vi "32_7_matrix_inverse.vi"(2 "n":i32, 3 "A":fxp<+/-,32,7>[](array[numeric])) -> (0 "divide by zero detected":bool, 1 "inv(A)":fxp<+/-,32,7>[](array[numeric]))   [LabVIEW 2020]
panel:
  in  "FXP_3":fxp<+,32,7>
  in  "FXP_2":fxp<+/-,32,7>=1.0 format="%#_32g"
  in  "FXP_1":fxp<+/-,32,7>
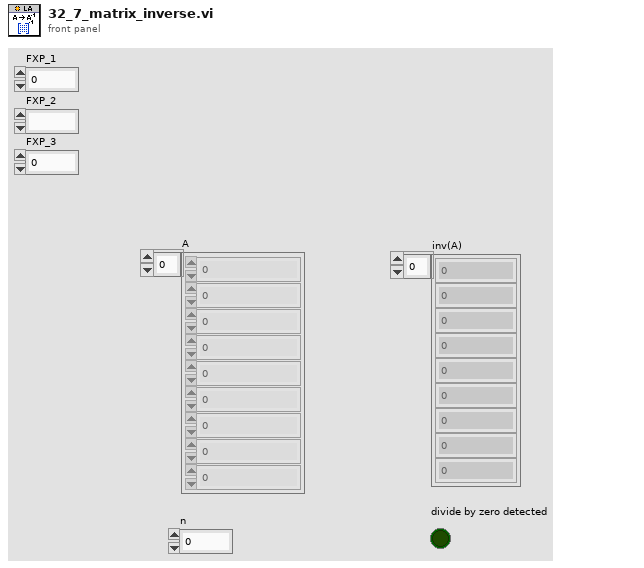
[diagram p1: front panel]
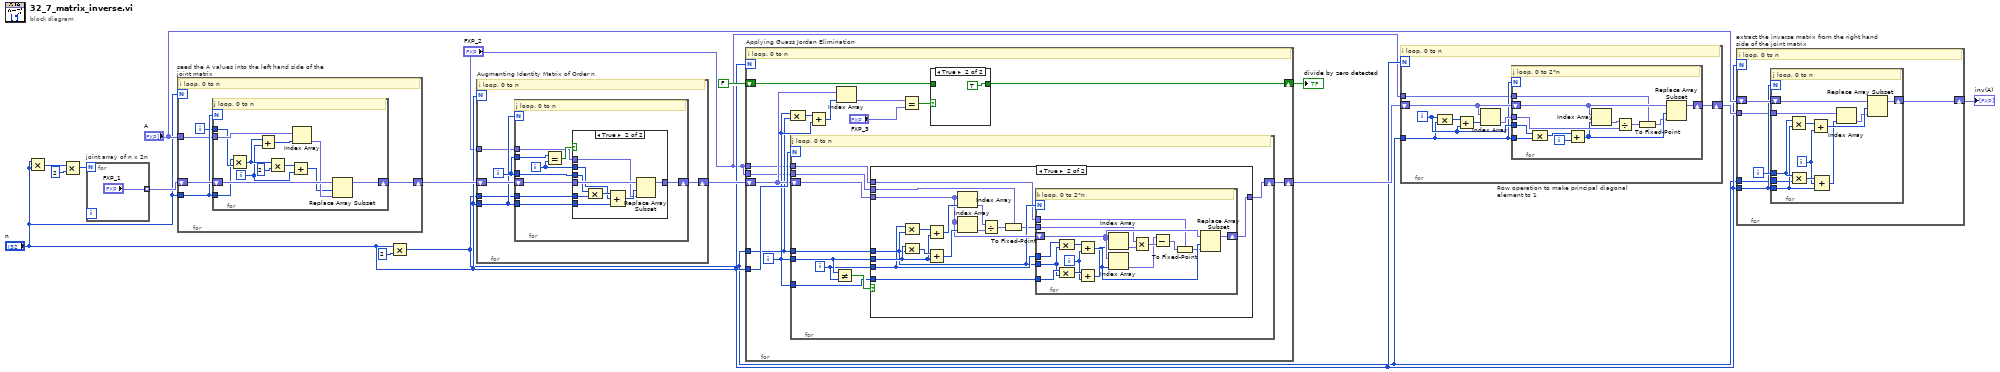
[diagram p0: block diagram]
diagram:
  n1 = Multiply(x="n", y="n") -> (x*y=w3:i32)
  n2 = Multiply(x=w3, y=2) -> (x*y=w6:i32)
  n3 = for "joint array of n x 2n" {
    N: w6 -> [_]
    tunnel: ["FXP_1"] -> w7 mode=indexing
  }
  n4 = for "seed the A values into the left hand side of the joint matrix" {
    N: "n" -> [_]
    shift-right: [w21] -> w8
    shift-left: w7 -> [w22]
    tunnel: "n" -> [w20]
    tunnel: "A" -> [w19]
    i -> [w18]
    # "i loop, 0 to n"
    n5 = for {
      N: w20 -> [_]
      shift-right: [w33] -> w21
      shift-left: w22 -> [w34]
      tunnel: w20 -> [w30]
      tunnel: w19 -> [w32]
      tunnel: w18 -> [w31]
      i -> [w24]
      # "j loop, 0 to n"
      n6 = Multiply(x=w30, y=w31) -> (x*y=w26:i32)
      n7 = Add(x=w26, y=w24) -> (x+y=w29:i32)
      n8 = Multiply(x=w26, y=2) -> (x*y=w25:i32)
      n9 = Add(x=w25, y=w24) -> (x+y=w23:i32)
      n10 = Index Array(array=w32, index=w29) -> (element=w28:fxp<+/-,32,7>)
      n11 = Replace Array Subset(array=w34, new element=w28, index=w23) -> (w33:fxp<+/-,32,7>[])
    }
  }
  n12 = Multiply(x="n", y=2) -> (x*y=w2:i32)
  n13 = for "Augmenting Identity Matrix of Order n" {
    N: "n" -> [_]
    shift-right: [w39] -> w11
    shift-left: w8 -> [w40]
    tunnel: "n" -> [w37]
    tunnel: w2 -> [w36]
    tunnel: "FXP_2" -> [w35]
    i -> [w38]
    # "i loop, 0 to n"
    n14 = for {
      N: w37 -> [_]
      tunnel: w38 -> [w49]
      shift-right: [w46] -> w39
      shift-left: w40 -> [w47]
      tunnel: w38 -> [w45]
      tunnel: w37 -> [w44]
      tunnel: w36 -> [w42]
      tunnel: w35 -> [w41]
      i -> [w43]
      # "j loop, 0 to n"
      n15 = Equal?(x=w49, y=w43) -> (x = y?=w48:bool)
      n16 = case shown="True" w48 {
        tunnel: w47 -> [w50 w59]
        tunnel: [w50 w57] -> w46
        tunnel: w45 -> [_ w58]
        tunnel: w44 -> [_ w54]
        tunnel: w43 -> [_ w55]
        tunnel: w42 -> [_ w52]
        tunnel: w41 -> [_ w51]
        frame False {
        }
        frame True {
          n17 = Compound Arithmetic op=MULTIPLY(w58, w52) -> (w56:i32)
          n18 = Compound Arithmetic op=ADD(w56, w55, w54) -> (w53:i32)
          n19 = Replace Array Subset(array=w59, new element=w51, index=w53) -> (w57:fxp<+/-,32,7>[])
        }
      }
    }
  }
  n20 = for "Applying Guass Jordan Elimination" {
    N: "n" -> [_]
    shift-right: [w67] -> w10
    shift-left: FALSE -> [w68]
    tunnel: "n" -> [w66]
    shift-right: [w63] -> w12
    shift-left: w11 -> [w65]
    tunnel: w2 -> [w62]
    tunnel: "FXP_2" -> [w61]
    tunnel: "FXP_2" -> [w60]
    i -> [w64]
    # "i loop, 0 to n"
    n21 = Compound Arithmetic op=MULTIPLY(w64, w62) -> (w72:i32)
    n22 = for {
      N: w66 -> [_]
      tunnel: w64 -> [w82]
      tunnel: w64 -> [w78]
      shift-right: [w77] -> w63
      shift-left: w65 -> [w81]
      tunnel: w62 -> [w76]
      tunnel: w61 -> [w75]
      tunnel: w60 -> [w74]
      i -> [w79]
      # "j loop, 0 to n"
      n23 = Not Equal?(x=w82, y=w79) -> (x != y?=w80:bool)
      n24 = case shown="True" w80 {
        tunnel: w82 -> [_ w93]
        tunnel: w81 -> [w83 w92]
        tunnel: w79 -> [_ w91]
        tunnel: w78 -> [_ w90]
        tunnel: [w83 w89] -> w77
        tunnel: w76 -> [_ w88]
        tunnel: w75 -> [_ w85]
        tunnel: w74 -> [_ w84]
        frame False {
        }
        frame True {
          n25 = Compound Arithmetic op=MULTIPLY(w91, w88) -> (w99:i32)
          n26 = Compound Arithmetic op=MULTIPLY(w93, w88) -> (w95:i32)
          n27 = Add(x=w99, y=w93) -> (x+y=w98:i32)
          n28 = Add(x=w95, y=w93) -> (x+y=w94:i32)
          n29 = Index Array(array=w92, index=w98) -> (element=w97:fxp<+/-,32,7>)
          n30 = Index Array(array=w92, index=w94) -> (element=w96:fxp<+/-,32,7>)
          n31 = Divide(x=w97, y=w96) -> (x/y=w87:fxp<+/-,64,33>)
          n32 = To Fixed-Point(fixed-point type=w85, number=w87) -> (fixed-point=w86:fxp<+/-,32,7>)
          n33 = for {
            N: w88 -> [_]
            tunnel: w91 -> [w115]
            tunnel: w86 -> [w111]
            tunnel: w90 -> [w108]
            shift-right: [w104] -> w89
            shift-left: w92 -> [w113]
            tunnel: w88 -> [w103]
            tunnel: w84 -> [w100]
            i -> [w109]
            # "k loop, 0 to 2*n"
            n34 = Compound Arithmetic op=MULTIPLY(w115, w103) -> (w116:i32)
            n35 = Compound Arithmetic op=MULTIPLY(w108, w103) -> (w110:i32)
            n36 = Add(x=w116, y=w109) -> (x+y=w114:i32)
            n37 = Add(x=w110, y=w109) -> (x+y=w107:i32)
            n38 = Index Array(array=w113, index=w107) -> (element=w112:fxp<+/-,32,7>)
            n39 = Index Array(array=w113, index=w114) -> (element=w105:fxp<+/-,32,7>)
            n40 = Multiply(x=w111, y=w112) -> (x*y=w106:fxp<+/-,64,14>)
            n41 = Subtract(x=w105, y=w106) -> (x-y=w102:fxp<+/-,64,14>)
            n42 = To Fixed-Point(fixed-point type=w100, number=w102) -> (fixed-point=w101:fxp<+/-,32,7>)
            n43 = Replace Array Subset(array=w113, new element=w101, index=w114) -> (w104:fxp<+/-,32,7>[])
          }
        }
      }
    }
    n44 = Add(x=w72, y=w64) -> (x+y=w71:i32)
    n45 = Index Array(array=w65, index=w71) -> (element=w70:fxp<+/-,32,7>)
    n46 = Equal?(x=w70, y="FXP_3") -> (x = y?=w69:bool)
    n47 = case shown="True" w69 {
      tunnel: w68 -> [w117 _]
      tunnel: [w117 TRUE] -> w67
      frame False {
      }
      frame True {
      }
    }
  }
  "divide by zero detected" <- w10
  n48 = for "Row operation to make principal diagonal element to 1" {
    N: "n" -> [_]
    shift-right: [w121] -> w15
    shift-left: w12 -> [w124]
    tunnel: w2 -> [w120]
    tunnel: "FXP_2" -> [w119]
    i -> [w123]
    # "i loop, 0 to n"
    n49 = Compound Arithmetic op=MULTIPLY(w123, w120) -> (w126:i32)
    n50 = Add(x=w126, y=w123) -> (x+y=w125:i32)
    n51 = Index Array(array=w124, index=w125) -> (element=w122:fxp<+/-,32,7>)
    n52 = for {
      N: w120 -> [_]
      tunnel: w123 -> [w138]
      tunnel: w122 -> [w134]
      shift-right: [w132] -> w121
      shift-left: w124 -> [w133]
      tunnel: w120 -> [w130]
      tunnel: w119 -> [w127]
      i -> [w136]
      # "j loop, 0 to 2*n"
      n53 = Compound Arithmetic op=MULTIPLY(w138, w130) -> (w137:i32)
      n54 = Add(x=w137, y=w136) -> (x+y=w131:i32)
      n55 = Index Array(array=w133, index=w131) -> (element=w135:fxp<+/-,32,7>)
      n56 = Divide(x=w135, y=w134) -> (x/y=w128:fxp<+/-,64,33>)
      n57 = To Fixed-Point(fixed-point type=w127, number=w128) -> (fixed-point=w129:fxp<+/-,32,7>)
      n58 = Replace Array Subset(array=w133, new element=w129, index=w131) -> (w132:fxp<+/-,32,7>[])
    }
  }
  n59 = for "extract the inverse matrix from the right hand side of the joint matrix" {
    N: "n" -> [_]
    tunnel: "n" -> [w141]
    shift-right: [w143] -> w14
    shift-left: "A" -> [w144]
    tunnel: w15 -> [w140]
    tunnel: w2 -> [w139]
    i -> [w142]
    # "i loop, 0 to n"
    n60 = for {
      N: w141 -> [_]
      shift-right: [w155] -> w143
      shift-left: w144 -> [w156]
      tunnel: w142 -> [w152]
      tunnel: w141 -> [w149]
      tunnel: w140 -> [w147]
      tunnel: w139 -> [w145]
      i -> [w150]
      # "j loop, 0 to n"
      n61 = Multiply(x=w152, y=w149) -> (x*y=w154:i32)
      n62 = Compound Arithmetic op=MULTIPLY(w152, w145) -> (w151:i32)
      n63 = Add(x=w154, y=w150) -> (x+y=w153:i32)
      n64 = Compound Arithmetic op=ADD(w151, w150, w149) -> (w148:i32)
      n65 = Index Array(array=w147, index=w148) -> (element=w146:fxp<+/-,32,7>)
      n66 = Replace Array Subset(array=w156, new element=w146, index=w153) -> (w155:fxp<+/-,32,7>[])
    }
  }
  "inv(A)" <- w14
